vi "Set SLSC Switch Description.vi"(8 "error in":errorcluster, 10 "description":string, 11 "slsc switch custom device in":T1 format="%.0x") -> (0 "error out":errorcluster, 3 "slsc switch custom device out":T1 format="%.0x")   [LabVIEW 2017, in "NI-SWITCH Scripting.lvlib"]
doc: "Sets the description for the SLSC Switch custom device."
uses:
  NI-SWITCH Scripting.lvlib
  <vilib>/NI VeriStand/Custom Device API/Custom Device API.lvlib
  <vilib>/NI Veristand/Custom Device API/Custom Device Item Ref.ctl
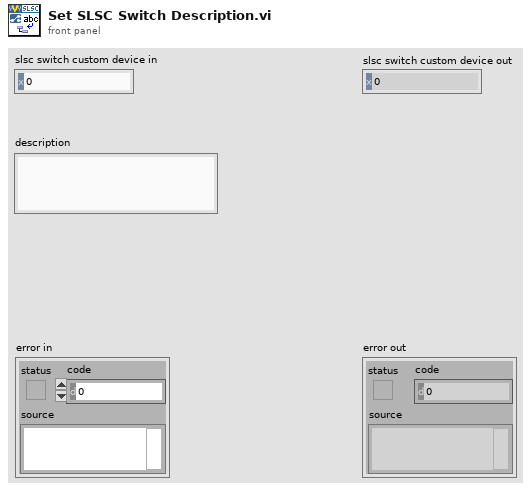
[diagram p1: front panel]
types:
  T1 = typedef "Custom Device API.lvlib/Custom Device Item Ref.ctl" = u64
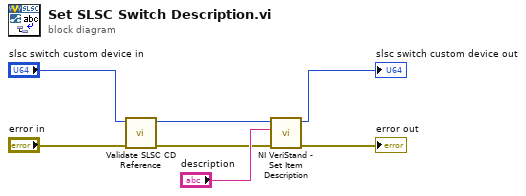
[diagram p0: block diagram]
diagram:
  n1 = call "Validate SLSC CD Reference.vi"("error in"="error in", "slsc switch custom device in"="slsc switch custom device in") -> ("error out"=w4:errorcluster, "slsc switch custom device out"=w2:T1)  [unwired: 8 in]
  n2 = call <vilib>:"NI VeriStand - Set Item Description.vi"("error in (no error)"=w4, "Description"="description", "Item Ref in"=w2) -> ("error out"=→"error out":errorcluster, "Item Ref out"=→"slsc switch custom device out":T1)  [unwired: 6 in, 1 out]
